vi "Script Add Custom Error -- Class.vi"(4 "Selection Owning Folder":path, 5 "Error Code":i32, 6 "Error Description":string, 7 "Error Name":string="TESTING.vi", 8 "error in":errorcluster, 9 "Error Arguments Window Ref":refnum<vi>, 10 "Project Reference":refnum<vi>, 11 "Class Ref":refnum<vi>) -> (0 "error out":errorcluster, 3 "Error VI Path":path)   [LabVIEW 2020, in "ConstantErrorsMaker.lvlib"]
uses:
  ConstantErrorsMaker.lvlib
  Selection Type--enum.ctl
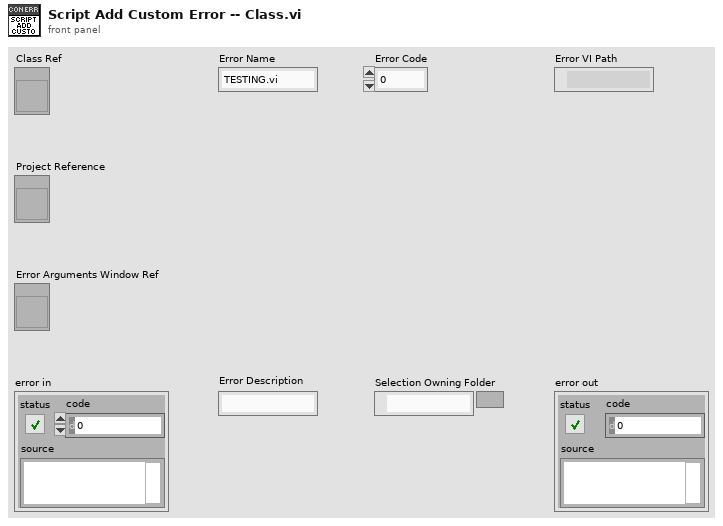
[diagram p1: front panel]
types:
  T1 = typedef "ConstantErrorsMaker.lvlib/Selection Type--enum.ctl" = enum16{"Project", "Library", "Class", "DQMH Singleton", "DQMH Cloneable"}
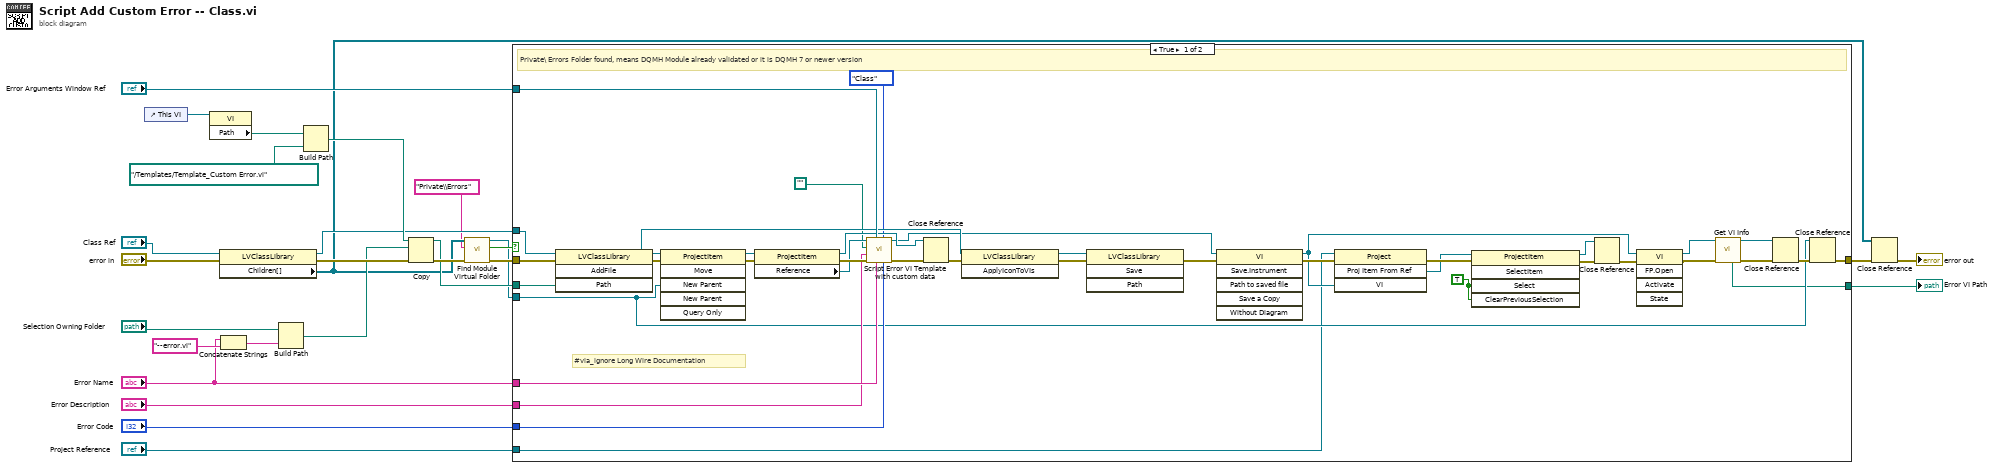
[diagram p0: block diagram]
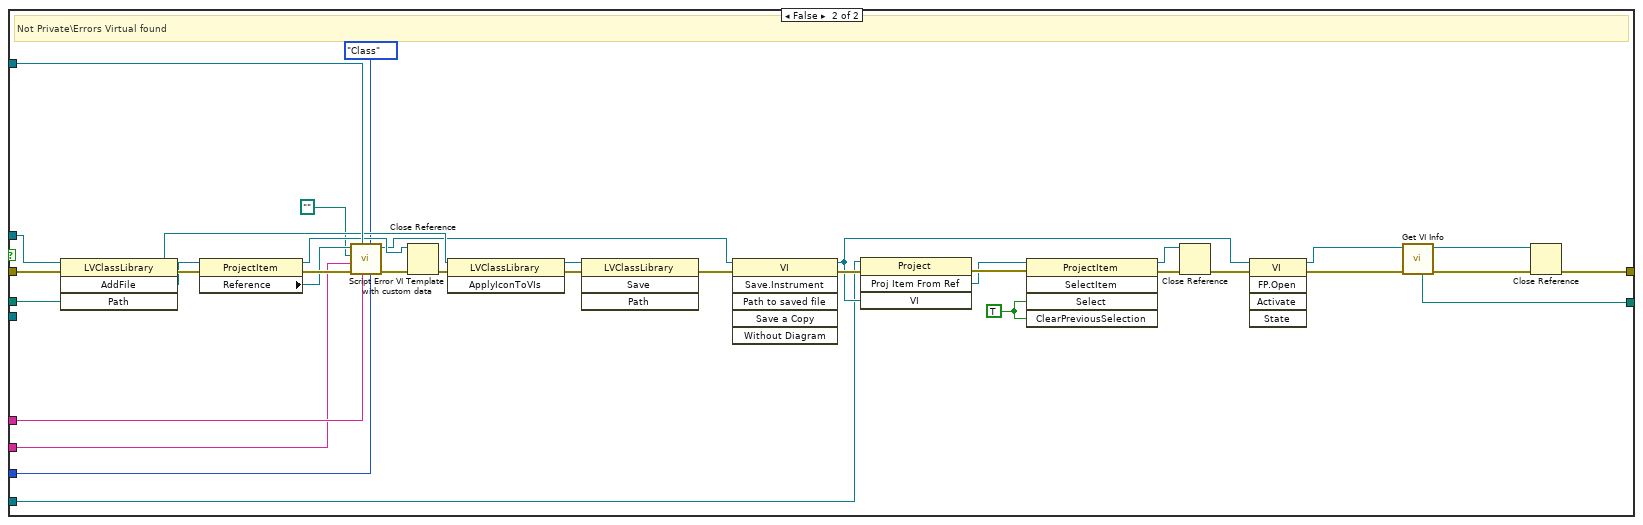
[diagram p2: hidden frame]
diagram:
  n1 = control-ref of="This VI"() -> (w19:refnum<vi>)
  n2 = property class="VI"(reference=w19) -> ("Path"=w18:path)  [unwired: 1 in, 2 out]
  n3 = property class="LVClassLibrary"(reference="Class Ref", error in="error in") -> (reference out=w15:refnum<vi>, error out=w22:errorcluster, "Children[]"=w8:refnum<vi>[])
  n4 = Concatenate Strings("Error Name", "--error.vi" ("input 1")) -> (w21:string)
  n5 = Build Path(base path="Selection Owning Folder", name or relative path=w21) -> (appended path=w20:path)
  n6 = Build Path(base path=w18, name or relative path=path "../Templates/Template_Custom Error.vi") -> (appended path=w16:path)
  n7 = Copy(8:w22, 10:w20, 11:w16) -> (0:w23:errorcluster, 3:w13:path)  [unwired: 2 in, 1 out]
  n8 = call "Find Module Virtual Folder.vi"("error in"=w23, "Virtual Folder"="Private\\Errors", "Children"=w8) -> ("error out"=w24:errorcluster, "Found?"=w7:bool, "ProjectItem out"=w6:refnum<vi>)  [unwired: 6 in]
  n9 = case shown="True" w7 {
    tunnel: [w65 w98] -> w27
    tunnel: w15 -> [w51 w89]
    tunnel: w13 -> [w52 w90]
    tunnel: "Error Name" -> [w45 w84]
    tunnel: "Error Code" -> [w48 w87]
    tunnel: "Error Arguments Window Ref" -> [w47 w86]
    tunnel: "Error Description" -> [w41 w80]
    tunnel: w6 -> [w40 _]
    tunnel: w24 -> [w59 w92]
    tunnel: "Project Reference" -> [w36 w76]
    tunnel: [w30 w70] -> w1
    frame True {
      w37 = TRUE ("Select")
      # "#via_ignore Long Wire Documentation"
      # "Private\\ Errors Folder found, means DQMH Module already validated or it is DQMH 7 or newer version"
      n10 = invoke class="LVClassLibrary" method="AddFile"(reference=w51, error in=w59, "Path"=w52) -> (reference out=w44:refnum<vi>, error out=w66:errorcluster, "AddFile"=w50:refnum<vi>)  [unwired: 1 in, 1 out]
      n11 = invoke class="ProjectItem" method="Move"(reference=w50, error in=w66, "New Parent"=w40) -> (reference out=w49:refnum<vi>, error out=w67:errorcluster)  [unwired: 3 in, 4 out]
      n12 = property class="ProjectItem"(reference=w49, error in=w67) -> (reference out=w46:refnum<vi>, error out=w53:errorcluster, "Reference"=w34:refnum<vi>)
      n13 = call "Script Error VI Template with custom data.vi"("Error Code"=w48, "Selection Type"=Selection_Type--enum."Class", "Error Name"=w45, "Error Arguments Window Ref"=w47, "error in"=w53, "Error Description"=w41, "Library Path"=path "", "VI Ref Error in"=w34) -> ("error out"=w55:errorcluster, "Custom Error VI Ref"=w42:refnum<vi>)  [unwired: 2 in]
      n14 = Close Reference(reference=w46, error in (no error)=w55) -> (error out=w64:errorcluster)
      n15 = invoke class="LVClassLibrary" method="ApplyIconToVIs"(reference=w44, error in=w64) -> (reference out=w43:refnum<vi>, error out=w63:errorcluster)  [unwired: 1 in, 1 out]
      n16 = invoke class="LVClassLibrary" method="Save"(reference=w43, error in=w63) -> (error out=w62:errorcluster)  [unwired: 2 in, 3 out]
      n17 = invoke class="VI" method="Save.Instrument"(reference=w42, error in=w62) -> (reference out=w39:refnum<vi>, error out=w58:errorcluster)  [unwired: 4 in, 4 out]
      n18 = invoke class="Project" method="Proj Item From Ref"(reference=w36, error in=w58, "VI"=w39) -> (error out=w57:errorcluster, "ProjItemFromRef"=w38:refnum<vi>)  [unwired: 1 in, 2 out]
      n19 = invoke class="ProjectItem" method="SelectItem"(reference=w38, error in=w57, "Select"=w37, "ClearPreviousSelection"=w37) -> (reference out=w35:refnum<vi>, error out=w56:errorcluster)  [unwired: 1 in, 3 out]
      n20 = Close Reference(reference=w35, error in (no error)=w56) -> (error out=w54:errorcluster)
      n21 = invoke class="VI" method="FP.Open"(reference=w39, error in=w54) -> (reference out=w32:refnum<vi>, error out=w61:errorcluster)  [unwired: 3 in, 3 out]
      n22 = call "Get VI Info.vi"("error in"=w61, "VI in"=w32) -> ("error out"=w33:errorcluster, "VI out"=w31:refnum<vi>, "VI Path"=w30:path)  [unwired: 4 in, 3 out]
      n23 = Close Reference(reference=w31, error in (no error)=w33) -> (error out=w60:errorcluster)
      n24 = Close Reference(reference=w40, error in (no error)=w60) -> (error out=w65:errorcluster)
    }
    frame False {
      w78 = TRUE ("Select")
      # "Not Private\\Errors Virtual found"
      n25 = invoke class="LVClassLibrary" method="AddFile"(reference=w89, error in=w92, "Path"=w90) -> (reference out=w83:refnum<vi>, error out=w103:errorcluster, "AddFile"=w88:refnum<vi>)  [unwired: 1 in, 1 out]
      n26 = property class="ProjectItem"(reference=w88, error in=w103) -> (reference out=w85:refnum<vi>, error out=w91:errorcluster, "Reference"=w74:refnum<vi>)
      n27 = call "Script Error VI Template with custom data.vi"("Error Code"=w87, "Selection Type"=Selection_Type--enum."Class", "Error Name"=w84, "Error Arguments Window Ref"=w86, "error in"=w91, "Error Description"=w80, "Library Path"=path "", "VI Ref Error in"=w74) -> ("error out"=w94:errorcluster, "Custom Error VI Ref"=w81:refnum<vi>)  [unwired: 2 in]
      n28 = Close Reference(reference=w85, error in (no error)=w94) -> (error out=w102:errorcluster)
      n29 = invoke class="LVClassLibrary" method="ApplyIconToVIs"(reference=w83, error in=w102) -> (reference out=w82:refnum<vi>, error out=w101:errorcluster)  [unwired: 1 in, 1 out]
      n30 = invoke class="LVClassLibrary" method="Save"(reference=w82, error in=w101) -> (error out=w100:errorcluster)  [unwired: 2 in, 3 out]
      n31 = invoke class="VI" method="Save.Instrument"(reference=w81, error in=w100) -> (reference out=w77:refnum<vi>, error out=w96:errorcluster)  [unwired: 4 in, 4 out]
      n32 = invoke class="Project" method="Proj Item From Ref"(reference=w76, error in=w96, "VI"=w77) -> (error out=w97:errorcluster, "ProjItemFromRef"=w79:refnum<vi>)  [unwired: 1 in, 2 out]
      n33 = invoke class="ProjectItem" method="SelectItem"(reference=w79, error in=w97, "Select"=w78, "ClearPreviousSelection"=w78) -> (reference out=w75:refnum<vi>, error out=w95:errorcluster)  [unwired: 1 in, 3 out]
      n34 = Close Reference(reference=w75, error in (no error)=w95) -> (error out=w93:errorcluster)
      n35 = invoke class="VI" method="FP.Open"(reference=w77, error in=w93) -> (reference out=w72:refnum<vi>, error out=w99:errorcluster)  [unwired: 3 in, 3 out]
      n36 = call "Get VI Info.vi"("error in"=w99, "VI in"=w72) -> ("error out"=w73:errorcluster, "VI out"=w71:refnum<vi>, "VI Path"=w70:path)  [unwired: 4 in, 3 out]
      n37 = Close Reference(reference=w71, error in (no error)=w73) -> (error out=w98:errorcluster)
    }
  }
  "Error VI Path" <- w1
  n38 = Close Reference(reference=w8, error in (no error)=w27) -> (error out=→"error out":errorcluster)
